vi "fgt set session Pressure Unit.vi"(8 "error in (no error)":errorcluster, 11 "unit":T1) -> (0 "error out":errorcluster)   [LabVIEW 2016, in "fgt_SDK.lvlib"]
doc: "Set pressure unit for all initialized channels, default value is \"mbar\". If type is invalid an error is returned.\nEvery pressure read value and sent command will then use this unit.\nExample of type: \"mbar\", \"millibar\", \"kPa\" ..."
uses:
  fgt_SDK.lvlib
  TypeDefs/fgt_PRESSURE_UNIT.ctl
  dlls/fgt_SDK_32.dll
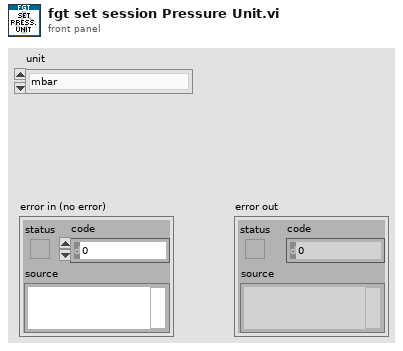
[diagram p1: front panel]
types:
  T1 = typedef "fgt_SDK.lvlib/fgt_PRESSURE_UNIT.ctl" = enum16{"mbar", "kPa", "PSI"}
  T2 = typedef "fgt_SDK.lvlib/fgt_STATUS_INFO.ctl" = cluster{"InstrType":T3, "instrSN":u16, "errorCode":u8, "infoCode":u8, "detail":string}
  T3 = typedef "fgt_SDK.lvlib/fgt_INSTRUMENT_TYPE.ctl" = enum32{"None", "MFCS", "MFCS_EZ", "FRP", "LineUP", "IPS"}
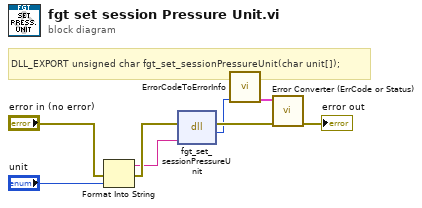
[diagram p0: block diagram]
diagram:
  # "DLL_EXPORT unsigned char fgt_set_sessionPressureUnit(char unit[]);"
  n1 = Format Into String(error in="error in (no error)", "unit") -> (resulting string=w3:string, error out=w4:errorcluster)  [unwired: 2 in]
  n2 = dll-call lib="C:/projects/SDK/fgt-sdk-labview/dlls/fgt_SDK_*.*" fn="fgt_set_sessionPressureUnit"(error in=w4, "unit"=w3) -> (error out=w8:errorcluster, "return type"=w2:u8)  [unwired: 3 in, 1 out]
  n3 = call "ErrorCodeToErrorInfo.vi"("return type"=w2) -> ("StatusInfo"=w1:T2)  [unwired: 10 in]
  n4 = call "Error Converter (ErrCode or Status).vi"("error in (no error)"=w8, "StatusInfo"=w1) -> ("error out"=→"error out":errorcluster)  [unwired: 9 in]
